vi "Write Enable.vi"(8 "error in (no error)":errorcluster, 10 "channel":refnum<class "TBM channel.lvclass">, 11 "SystemLink File configuration in":refnum<class "SystemLink File configuration.lvclass">) -> (0 "error out":errorcluster, 3 "SystemLink File configuration out":refnum<class "SystemLink File configuration.lvclass">)   [LabVIEW 2015, in "SystemLink File configuration.lvclass"]
uses:
  SystemLink File configuration.lvclass
  <vilib>/NI/Tag Bus Module Framework/channel/TBM channel.lvclass
  SystemLink File configuration.lvclass/SystemLink File configuration.ctl
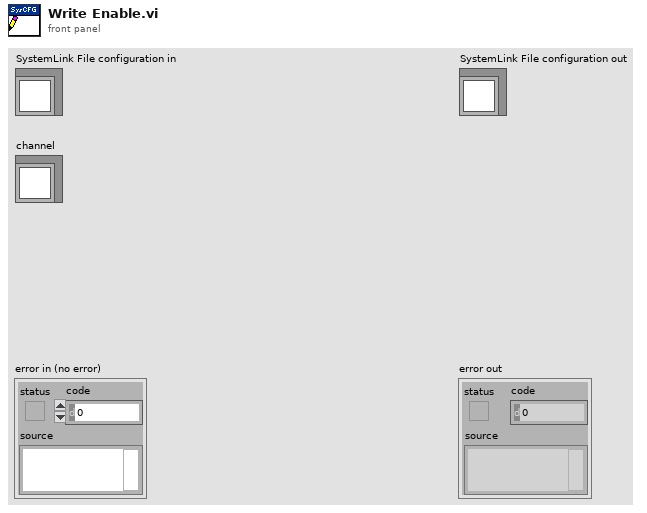
[diagram p1: front panel]
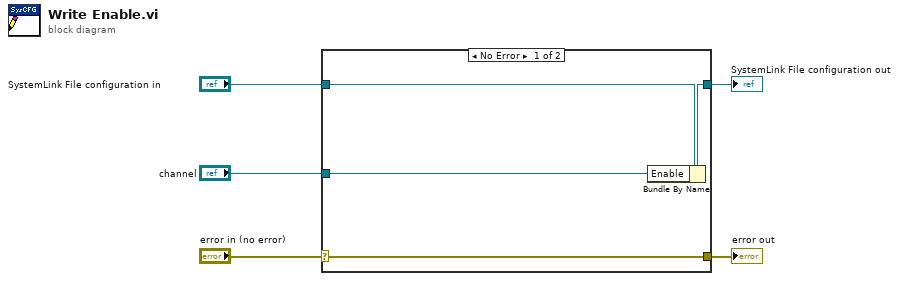
[diagram p0: block diagram]
diagram:
  n1 = case shown="No Error" "error in (no error)" {
    selector: "error in (no error)" -> [w9 w10]
    tunnel: [w9 w10] -> w4
    tunnel: [w7 w11] -> w2
    tunnel: "SystemLink File configuration in" -> [w8 w11]
    tunnel: "channel" -> [w6 _]
    frame No Error {
      n2 = Bundle By Name(cluster=w8, "Enable"=w6) -> (w7:refnum<class "SystemLink File configuration.lvclass">)
    }
    frame Error {
    }
  }
  "error out" <- w4
  "SystemLink File configuration out" <- w2
